vi "color_detector.vi"(11 "return type in":string) -> (3 "return type out":string[](array[string]))   [LabVIEW 2019]
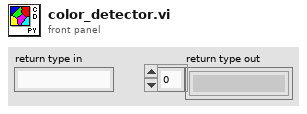
[diagram p1: front panel]
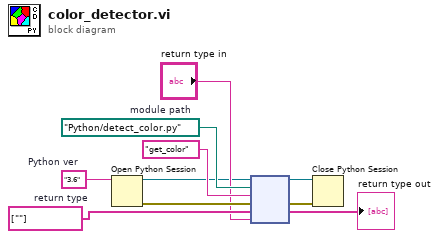
[diagram p0: block diagram]
diagram:
  w9 = string[] [""]  # return type
  w6 = "3.6"  # Python ver
  w7 = path "Python/detect_color.py"  # module path
  n1 = Open Python Session(python version=w6) -> (session out=w1:refnum<k35>, error out=w8:errorcluster)  [unwired: 2 in]
  n2 = node(w1, w7, "get_color" ("time format string (%c)"), w8, w9, "return type in") -> (w2:refnum<k35>, w3:errorcluster, →"return type out":string[])  [unwired: 1 in, 2 out]
  n3 = Close Python Session(session in=w2, error in=w3) -> ()  [unwired: 1 out]
